vi "FRA.vi"(0 "LoadProcedure":refnum<k24>, 1 "stop":refnum<vi>, 7 "error in":errorcluster) -> (18 "Bode phase":cluster{"Y":dbl[], "Y":dbl[]}[](graph), 19 "Bode Z":cluster{"Y":dbl[], "Y":dbl[]}[](graph), 20 "Nyquist":cluster{"Y":dbl[], "Y":dbl[]}[](graph), 21 "E & I":cluster{"Y":dbl[], "Y":dbl[]}[](graph), 22 "-Phase":dbl[](array[numeric]), 23 "Frequency":dbl[](array[numeric]), 24 "-Z''":dbl[](array[numeric]), 25 "Z":dbl[](array[numeric]), 26 "Z'":dbl[](array[numeric]), 27 "error out":errorcluster)   [LabVIEW 2014]
doc: "Shows the Frequency Response Analysis measured values from the instrument."
uses:
  H:/Program Files/Metrohm Autolab/Autolab SDK 2.0/EcoChemie.Autolab.Sdk.dll
  EcoChemie.Autolab.Sdk.dll
  H:/Program Files/Metrohm Autolab/Autolab SDK 2.0/EcoChemie100.dll
  EcoChemie100.dll
panel:
  out "Event":bool
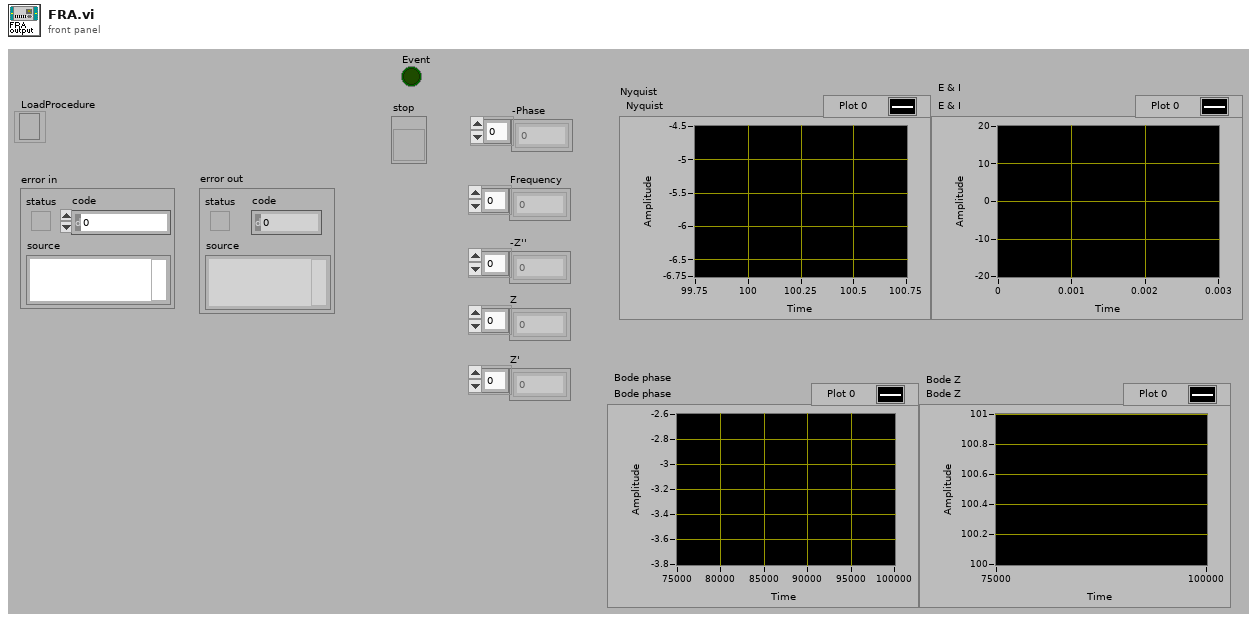
[diagram p1: front panel]
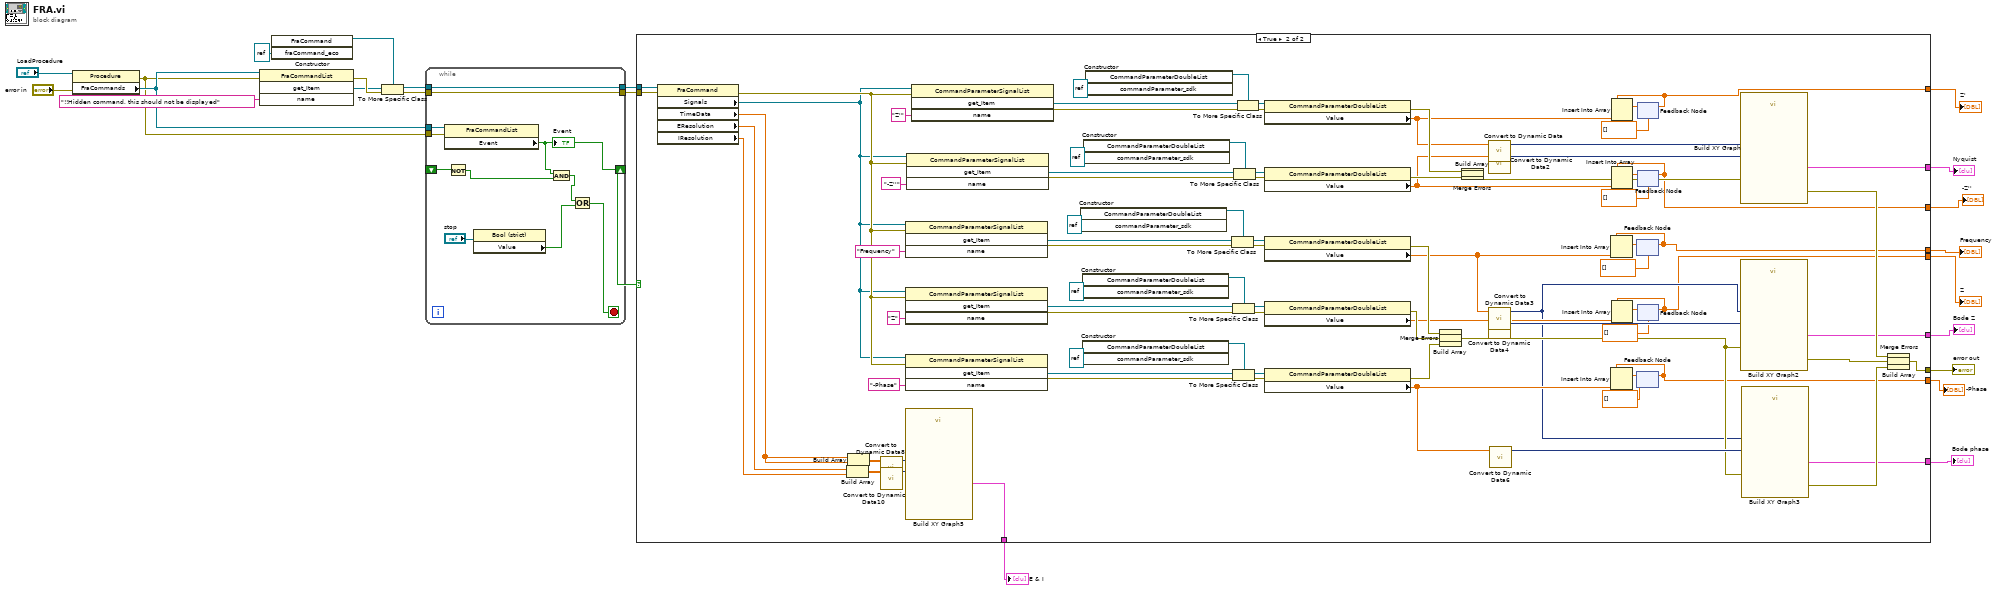
[diagram p0: block diagram]
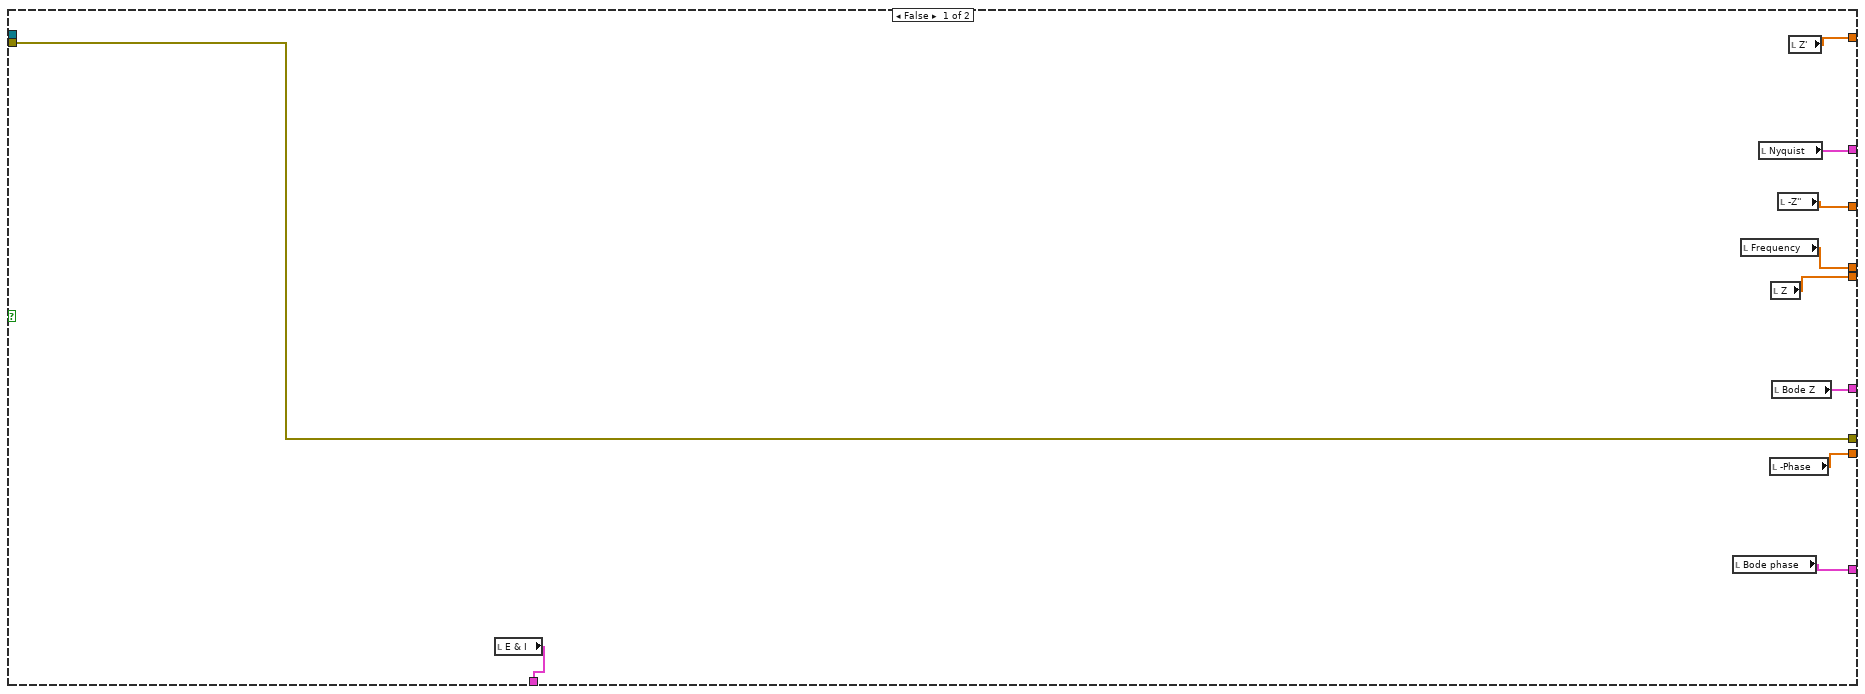
[diagram p2: hidden frame]
diagram:
  n1 = property class="Procedure"(reference="LoadProcedure", error in="error in") -> (error out=w17:errorcluster, "FraCommands"=w18:refnum<k24>)  [unwired: 1 out]
  n2 = invoke class="FraCommandList" method="get_Item"(reference=w18, error in=w17, "name"="!!Hidden command, this should not be displayed" ("Fra Commands")) -> (error out=w21:errorcluster, "get_Item"=w20:refnum<k24>)  [unwired: 1 in, 2 out]
  n3 = constructor class="FraCommand"("fraCommand_eco"=refnum<k24> refnum) -> (reference out=w22:refnum<k24>)  [unwired: 3 in, 3 out]
  n4 = To More Specific Class(target class=w22, reference=w20, error in=w21) -> (specific class reference=w3:refnum<k24>, error out=w5:errorcluster)
  n5 = while {
    tunnel: w18 -> [w35]
    tunnel: w17 -> [w34]
    shift-right: [w32] -> w7
    shift-left: _ -> [w33]
    tunnel: [w28] -> w6
    tunnel: w5 -> [w28]
    tunnel: [w27] -> w4
    tunnel: w3 -> [w27]
    stop <- w29 stop-if-true
    n6 = property class="FraCommandList"(reference=w35, error in=w34) -> ("Event"=w32:bool)  [unwired: 2 out]
    "Event" <- w32
    n7 = Not(x=w33) -> (.not. x?=w31:bool)
    n8 = property class="Bool (strict)"(reference="stop") -> ("Value"=w25:bool)  [unwired: 1 in, 2 out]
    n9 = And(x=w32, y=w31) -> (x .and. y?=w30:bool)
    n10 = Or(x=w30, y=w25) -> (x .or. y?=w29:bool)
  }
  n11 = case shown="True" w7 {
    tunnel: [w45 w134] -> w24
    tunnel: w4 -> [_ w133]
    tunnel: w6 -> [w45 w132]
    tunnel: [w41 w62] -> w16
    tunnel: [w42 w61] -> w15
    tunnel: [w43 w60] -> w14
    tunnel: [w44 w59] -> w13
    tunnel: [w36 w58] -> w12
    tunnel: [w37 w57] -> w11
    tunnel: [w38 w56] -> w10
    tunnel: [w39 w55] -> w9
    tunnel: [w40 w54] -> w8
    frame False {
      n12 = local read "E & I"() -> (w44:cluster{"Y":dbl[], "Y":dbl[]}[])
      n13 = local read "Bode phase"() -> (w43:cluster{"Y":dbl[], "Y":dbl[]}[])
      n14 = local read "Frequency"() -> (w38:dbl[])
      n15 = local read "Nyquist"() -> (w41:cluster{"Y":dbl[], "Y":dbl[]}[])
      n16 = local read "-Phase"() -> (w36:dbl[])
      n17 = local read "Z"() -> (w37:dbl[])
      n18 = local read "Bode Z"() -> (w42:cluster{"Y":dbl[], "Y":dbl[]}[])
      n19 = local read "-Z''"() -> (w39:dbl[])
      n20 = local read "Z'"() -> (w40:dbl[])
    }
    frame True {
      n21 = property class="FraCommand"(reference=w133, error in=w132) -> (error out=w106:errorcluster, "Signals"=w105:refnum<k24>, "TimeData"=w66:dbl[], "EResolution"=w65:dbl[], "IResolution"=w64:dbl[])  [unwired: 1 out]
      n22 = Build Array(w65, w64) -> (w91:dbl[][])
      n23 = Build Array(w66, w66) -> (w89:dbl[][])
      n24 = call "Convert to Dynamic Data8"("2D Array"=w89) -> ("Dynamic Data Type"=w88:dynamicdata)  [unwired: 3 in]
      n25 = call "Convert to Dynamic Data10"("2D Array"=w91) -> ("Dynamic Data Type"=w90:dynamicdata)  [unwired: 3 in]
      n26 = invoke class="CommandParameterSignalList" method="get_Item"(reference=w105, error in=w106, "name"="Frequency") -> (error out=w116:errorcluster, "get_Item"=w115:refnum<k24>)  [unwired: 1 in, 2 out]
      n27 = invoke class="CommandParameterSignalList" method="get_Item"(reference=w105, error in=w106, "name"="Z") -> (error out=w121:errorcluster, "get_Item"=w120:refnum<k24>)  [unwired: 1 in, 2 out]
      n28 = invoke class="CommandParameterSignalList" method="get_Item"(reference=w105, error in=w106, "name"="-Phase") -> (error out=w111:errorcluster, "get_Item"=w110:refnum<k24>)  [unwired: 1 in, 2 out]
      n29 = call "Build XY Graph5"("Y Input"=w90, "X Input"=w88) -> ("XY Graph"=w59:cluster{"Y":dbl[], "Y":dbl[]}[])  [unwired: 8 in, 1 out]
      n30 = invoke class="CommandParameterSignalList" method="get_Item"(reference=w105, error in=w106, "name"="-Z''") -> (error out=w131:errorcluster, "get_Item"=w130:refnum<k24>)  [unwired: 1 in, 2 out]
      n31 = invoke class="CommandParameterSignalList" method="get_Item"(reference=w105, error in=w106, "name"="Z'") -> (error out=w126:errorcluster, "get_Item"=w125:refnum<k24>)  [unwired: 1 in, 2 out]
      n32 = constructor class="CommandParameterDoubleList"("commandParameter_sdk"=refnum<k24> refnum) -> (reference out=w114:refnum<k24>)  [unwired: 3 in, 3 out]
      n33 = constructor class="CommandParameterDoubleList"("commandParameter_sdk"=refnum<k24> refnum) -> (reference out=w119:refnum<k24>)  [unwired: 3 in, 3 out]
      n34 = constructor class="CommandParameterDoubleList"("commandParameter_sdk"=refnum<k24> refnum) -> (reference out=w109:refnum<k24>)  [unwired: 3 in, 3 out]
      n35 = constructor class="CommandParameterDoubleList"("commandParameter_sdk"=refnum<k24> refnum) -> (reference out=w129:refnum<k24>)  [unwired: 3 in, 3 out]
      n36 = constructor class="CommandParameterDoubleList"("commandParameter_sdk"=refnum<k24> refnum) -> (reference out=w124:refnum<k24>)  [unwired: 3 in, 3 out]
      n37 = To More Specific Class(target class=w114, reference=w115, error in=w116) -> (specific class reference=w113:refnum<k24>, error out=w112:errorcluster)
      n38 = To More Specific Class(target class=w119, reference=w120, error in=w121) -> (specific class reference=w118:refnum<k24>, error out=w117:errorcluster)
      n39 = To More Specific Class(target class=w109, reference=w110, error in=w111) -> (specific class reference=w108:refnum<k24>, error out=w107:errorcluster)
      n40 = To More Specific Class(target class=w129, reference=w130, error in=w131) -> (specific class reference=w128:refnum<k24>, error out=w127:errorcluster)
      n41 = To More Specific Class(target class=w124, reference=w125, error in=w126) -> (specific class reference=w123:refnum<k24>, error out=w122:errorcluster)
      n42 = property class="CommandParameterDoubleList"(reference=w123, error in=w122) -> (error out=w92:errorcluster, "Value"=w82:dbl[])  [unwired: 1 out]
      n43 = property class="CommandParameterDoubleList"(reference=w128, error in=w127) -> (error out=w93:errorcluster, "Value"=w81:dbl[])  [unwired: 1 out]
      n44 = property class="CommandParameterDoubleList"(reference=w113, error in=w112) -> (error out=w97:errorcluster, "Value"=w85:dbl[])  [unwired: 1 out]
      n45 = property class="CommandParameterDoubleList"(reference=w118, error in=w117) -> (error out=w96:errorcluster, "Value"=w84:dbl[])  [unwired: 1 out]
      n46 = property class="CommandParameterDoubleList"(reference=w108, error in=w107) -> (error out=w95:errorcluster, "Value"=w83:dbl[])  [unwired: 1 out]
      n47 = Build Array(w97, w96, w95) -> (w48:errorcluster[])
      n48 = Merge Errors(w48) -> (w80:errorcluster)
      n49 = Build Array(w92, w93) -> (w47:errorcluster[])
      n50 = Merge Errors(w47) -> (w94:errorcluster)
      n51 = call "Convert to Dynamic Data"("Array"=w82) -> ("Dynamic Data Type"=w99:dynamicdata)  [unwired: 3 in]
      n52 = call "Convert to Dynamic Data2"("Array"=w81) -> ("Dynamic Data Type"=w98:dynamicdata)  [unwired: 3 in]
      n53 = call "Convert to Dynamic Data3"("Array"=w85) -> ("Dynamic Data Type"=w63:dynamicdata)  [unwired: 3 in]
      n54 = call "Convert to Dynamic Data4"("Array"=w84) -> ("Dynamic Data Type"=w87:dynamicdata)  [unwired: 3 in]
      n55 = call "Convert to Dynamic Data6"("Array"=w83) -> ("Dynamic Data Type"=w86:dynamicdata)  [unwired: 3 in]
      n56 = feedback #1(dbl[] []) -> (w56:dbl[])
      n57 = Insert Into Array(array=w56, new element=w85) -> (w76:dbl[])  [unwired: 1 in]
      n58 = feedback-in #1(w76) -> ()
      n59 = feedback #2(dbl[] []) -> (w58:dbl[])
      n60 = Insert Into Array(array=w58, new element=w83) -> (w74:dbl[])  [unwired: 1 in]
      n61 = feedback-in #2(w74) -> ()
      n62 = feedback #3(dbl[] []) -> (w54:dbl[])
      n63 = Insert Into Array(array=w54, new element=w82) -> (w73:dbl[])  [unwired: 1 in]
      n64 = feedback-in #3(w73) -> ()
      n65 = feedback #4(dbl[] []) -> (w55:dbl[])
      n66 = Insert Into Array(array=w55, new element=w81) -> (w72:dbl[])  [unwired: 1 in]
      n67 = feedback-in #4(w72) -> ()
      n68 = feedback #5(dbl[] []) -> (w57:dbl[])
      n69 = Insert Into Array(array=w57, new element=w84) -> (w75:dbl[])  [unwired: 1 in]
      n70 = feedback-in #5(w75) -> ()
      n71 = call "Build XY Graph"("error in (no error)"=w94, "Y Input"=w98, "X Input"=w99) -> ("error out"=w78:errorcluster, "XY Graph"=w62:cluster{"Y":dbl[], "Y":dbl[]}[])  [unwired: 7 in]
      n72 = call "Build XY Graph2"("error in (no error)"=w80, "Y Input"=w87, "X Input"=w63) -> ("error out"=w79:errorcluster, "XY Graph"=w61:cluster{"Y":dbl[], "Y":dbl[]}[])  [unwired: 7 in]
      n73 = call "Build XY Graph3"("error in (no error)"=w80, "Y Input"=w86, "X Input"=w63) -> ("error out"=w77:errorcluster, "XY Graph"=w60:cluster{"Y":dbl[], "Y":dbl[]}[])  [unwired: 7 in]
      n74 = Build Array(w78, w79, w77) -> (w46:errorcluster[])
      n75 = Merge Errors(w46) -> (w134:errorcluster)
    }
  }
  "error out" <- w24
  "Nyquist" <- w16
  "Bode Z" <- w15
  "Bode phase" <- w14
  "E & I" <- w13
  "Z'" <- w8
  "-Z''" <- w9
  "Frequency" <- w10
  "Z" <- w11
  "-Phase" <- w12
